vi "Tell Self.vi"(4 "Priority":bool, 7 "Actor in":refnum<class "Actor.lvclass">, 8 "Error in":errorcluster, 9 "Error":errorcluster, 10 "Unified Actor":refnum<class "Actor.lvclass">) -> (0 "Error out":errorcluster, 5 "Actor out":refnum<class "Actor.lvclass">)   [LabVIEW 2020, in "jettl.lvlib" / "Stopped jettl Msg.lvlib" / "Stopped.lvlib"]
uses:
  Stopped.lvlib
  Actor/Actor.lvclass
  jettl.lvlib
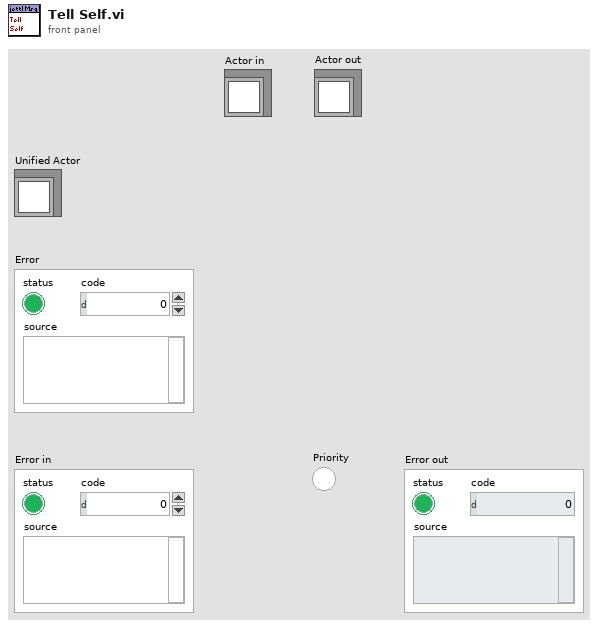
[diagram p1: front panel]
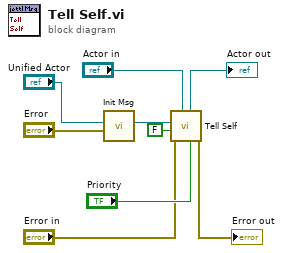
[diagram p0: block diagram]
diagram:
  n1 = call "Init Msg.vi"("Error"="Error", "Unified Actor"="Unified Actor") -> ("Msg"=w1:refnum<class "Msg.lvclass">)  [unwired: 9 in]
  n2 = call "Tell Self.vi"("Priority"="Priority", "Actor in"="Actor in", "Error in"="Error in", "Reply"=FALSE, "Msg"=w1) -> ("Error out"=→"Error out":errorcluster, "Actor out"=→"Actor out":refnum<class "Actor.lvclass">)  [unwired: 5 in]
